vi "Write_parameter.vi"(8 "error in (no error)":errorcluster caption="entrée d'erreur (pas d'erreur)", 10 "Parameter":string, 11 "Class Instrument Power_Supply en entrée":refnum<class "Class Instrument Power_Supply.lvclass">) -> (0 "error out":errorcluster caption="sortie d'erreur", 3 "Class Instrument Power_Supply en sortie":refnum<class "Class Instrument Power_Supply.lvclass">)   [LabVIEW 2020, in "Library Instrument & Equipement.lvlib" / "Library Instruments.lvlib" / "Class Instrument Power_Supply.lvclass"]
uses:
  Class Instrument Power_Supply.lvclass
  Commun VI/TypeDef/Command Power_Supply/Parameter Power_Supply.ctl
  Power_Supply/Power_Supply (Default)/Power_Supply (Default).lvclass
  JSON API/JSON Value/Set from JSON string.vi
  Instrument (Default)/Class Instrument (Default).lvclass
  JSON API/JSON Value/JSON Value.lvclass
  Class Instrument Power_Supply.lvclass/Class Instrument Power_Supply.ctl
  JSON API/Variant JSON/Variant JSON.lvlib
  JSON API/Get Polymorphic/JSON GetSet.lvlib
  Commun VI/Library Commun.lvlib
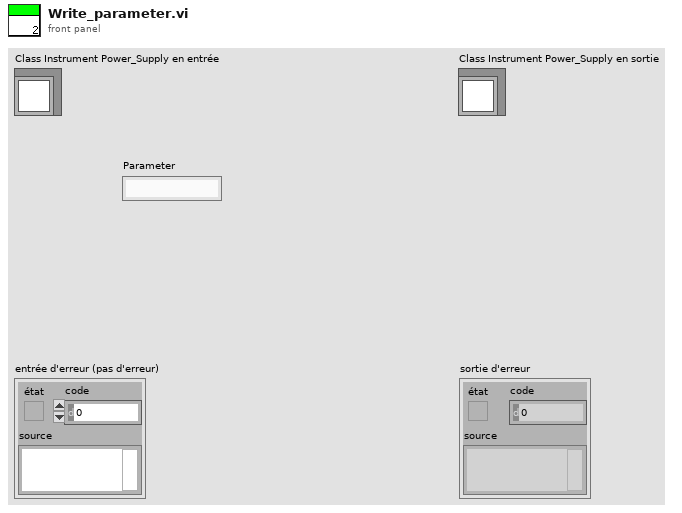
[diagram p1: front panel]
types:
  T1 = typedef "Library Commun.lvlib/Parameter Power_Supply.ctl" = cluster{"Device_Addr":refnum<visa-resource-name>, "Current":dbl, "Channel":i32, "Voltage":dbl, " Class Power_Supply":refnum<class "Power_Supply (Default).lvclass">}
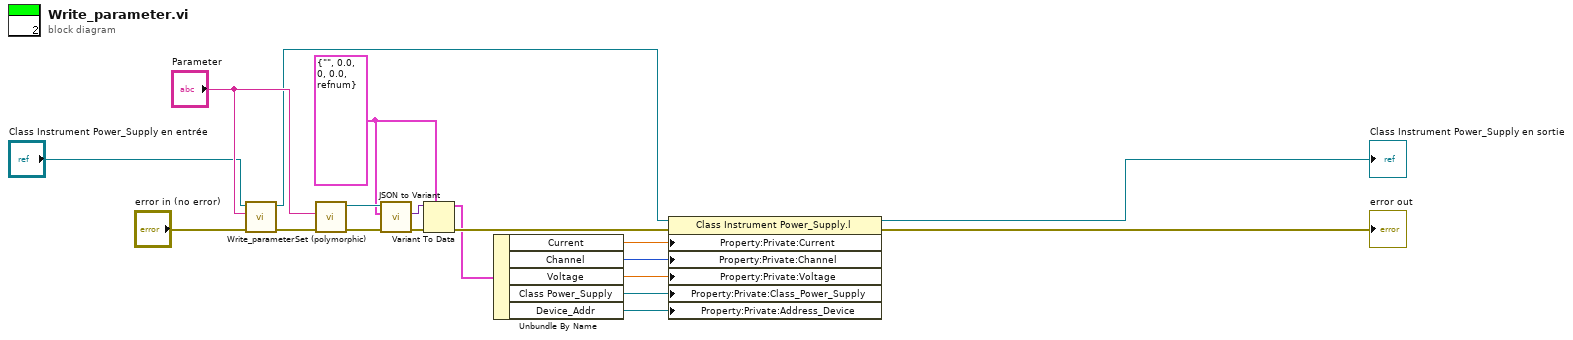
[diagram p0: block diagram]
diagram:
  w10 = T1 {"Device_Addr"="", "Current"=0.0, "Channel"=0, "Voltage"=0.0, " Class Power_Supply"=refnum} ("Parameter")
  n1 = call-parent "Write_parameter.vi"("error in (no error)"="error in (no error)", "Parameter"="Parameter", "Class Instrument (Default) en entrée"="Class Instrument Power_Supply en entrée") -> ("error out"=w9:errorcluster, "Class Instrument (Default) en sortie"=w6:refnum<class "Class Instrument Power_Supply.lvclass">)  [unwired: 7 in]
  n2 = call-poly "Set (polymorphic).vi"("error in (no error)"=w9, "JSON stream"="Parameter") -> ("error out"=w17:errorcluster, "JSON Value out"=w19:refnum<class "JSON Value.lvclass">)  [unwired: 7 in, 1 out]
  n3 = call "JSON to Variant.vi"("error in (no error)"=w17, "Variant (Data Type)"=w10, "JSON Value"=w19) -> ("error out"=w18:errorcluster, "Variant out"=w16:variant)  [unwired: 7 in]
  n4 = Variant To Data(error in=w18, type=w10, Variant=w16) -> (data=w4:T1, error out=w14:errorcluster)
  n5 = Unbundle By Name(w4) -> ("Current"=w11:dbl, "Channel"=w12:i32, "Voltage"=w13:dbl, "Class Power_Supply"=w5:refnum<class "Power_Supply (Default).lvclass">, "Device_Addr"=w1:refnum<visa-resource-name>)
  n6 = property class="Class Instrument Power_Supply.l"(reference=w6, error in=w14, "Property:Private:Current"=w11, "Property:Private:Channel"=w12, "Property:Private:Voltage"=w13, "Property:Private:Class_Power_Supply"=w5, "Property:Private:Address_Device"=w1) -> (reference out=→"Class Instrument Power_Supply en sortie":refnum<class "Class Instrument Power_Supply.lvclass">, error out=→"error out":errorcluster)
